vi "svx_Channel Type to Sensor Type String.vi"(3 "channel type":T1 items=["Voltage (V)"=0, "Charge (C)"=9, "-"=99, "SPL (Pa)"=3, "Force (lbf)"=6, "Force (N)"=1, "Acceleration (g) - IEPE"=2, "Acceleration (g) - Charge"=12, "Acceleration (g) - 4 wire DC Voltage"=22, "Velocity (in/s)"=7, "Velocity (mm/s)"=8, "Prox Probe (mil)"=4, "Prox Probe (mm)"=5]) -> (1 "sensor type":string)   [LabVIEW 2017, in "SVX NI-DAQmx AI Configuration XControl.xctl"]
uses:
  <vilib>/addons/Sound and Vibration/svt_DAQmx/Configuration XControl/SVX NI-DAQmx AI Configuration XControl.xctl
  <vilib>/addons/Sound and Vibration/svt_DAQmx/Configuration XControl/Controls/svx_DAQ_ChannelType.ctl
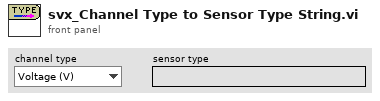
[diagram p1: front panel]
types:
  T1 = typedef "SVX NI-DAQmx AI Configuration XControl.xctl/svx_DAQ_ChannelType.ctl" = u16
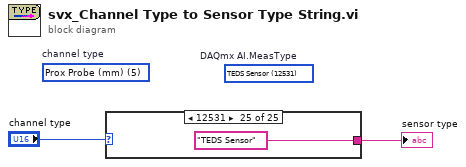
[diagram p0: block diagram]
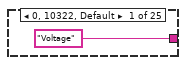
[diagram p2: hidden frame]
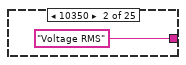
[diagram p3: hidden frame]
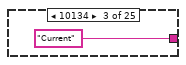
[diagram p4: hidden frame]
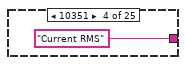
[diagram p5: hidden frame]
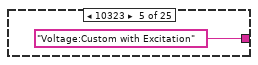
[diagram p6: hidden frame]
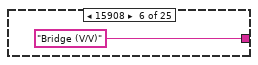
[diagram p7: hidden frame]
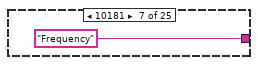
[diagram p8: hidden frame]
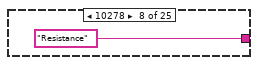
[diagram p9: hidden frame]
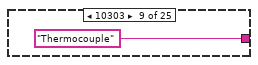
[diagram p10: hidden frame]
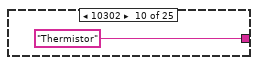
[diagram p11: hidden frame]
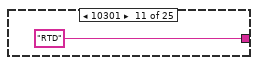
[diagram p12: hidden frame]
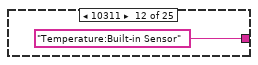
[diagram p13: hidden frame]
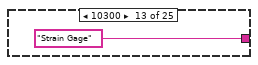
[diagram p14: hidden frame]
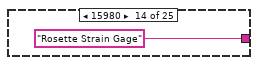
[diagram p15: hidden frame]
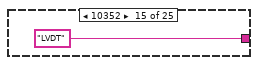
[diagram p16: hidden frame]
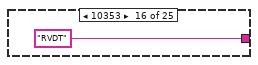
[diagram p17: hidden frame]
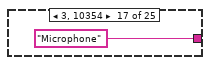
[diagram p18: hidden frame]
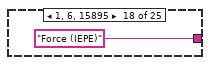
[diagram p19: hidden frame]
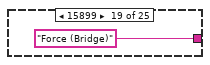
[diagram p20: hidden frame]
diagram:
  (unwired) T1 5 items=["Voltage (V)"=0, "SPL (Pa)"=3, "Force (lbf)"=6, "Force (N)"=1, "Acceleration (g)"=2, "Velocity (in/s)"=7, "Velocity (mm/s)"=8, "Prox Probe (mil)"=4, "Prox Probe (mm)"=5]  # channel type
  (unwired) 12531 items=["Voltage"=10322, "Voltage RMS"=10350, "Current"=10134, "Current RMS"=10351, "More:Voltage:Custom with Excitation"=10323, "More:Bridge (V/V)"=15908, "Frequency"=10181, "Resistance"=10278, "Temperature:Thermocouple"=10303, "Temperature:Thermistor"=10302, "Temperature:RTD"=10301, "Temperature:Built-in Sensor"=10311, "Strain Gage"=10300, "Rosette Strain Gage"=15980, "Position:LVDT"=10352, "Position:RVDT"=10353, "Position:Eddy Current Proximity Probe"=14835, "Accelerometer"=10356, "Velocity:IEPE Sensor"=15966, "Force:Bridge"=15899, "Force:IEPE Sensor"=15895, "Pressure:Bridge"=15902, "Sound Pressure:Microphone"=10354, "Torque:Bridge"=15905, "TEDS Sensor"=12531]  # DAQmx AI.MeasType
  n1 = case shown="12531" "channel type" {
    tunnel: ["Voltage" "Voltage RMS" "Current" "Current RMS" "Voltage:Custom with Excitation" "Bridge (V/V)" "Frequency" "Resistance" "Thermocouple" "Thermistor" "RTD" "Temperature:Built-in Sensor" "Strain Gage" "Rosette Strain Gage" "LVDT" "RVDT" "Microphone" "Force (IEPE)" "Force (Bridge)" "Pressure (Bridge)" "Torque (Bridge)" "Accelerometer" "Velocity (IEPE)" "Proximity Probe" "TEDS Sensor"] -> w2
    frame 0, 10322, Default {
    }
    frame 10350 {
    }
    frame 10134 {
    }
    frame 10351 {
    }
    frame 10323 {
    }
    frame 15908 {
    }
    frame 10181 {
    }
    frame 10278 {
    }
    frame 10303 {
    }
    frame 10302 {
    }
    frame 10301 {
    }
    frame 10311 {
    }
    frame 10300 {
    }
    frame 15980 {
    }
    frame 10352 {
    }
    frame 10353 {
    }
    frame 3, 10354 {
    }
    frame 1, 6, 15895 {
    }
    frame 15899 {
    }
    frame 15902 {
    }
    frame 15905 {
    }
    frame 2, 10356 {
    }
    frame 7, 8, 15966 {
    }
    frame 4, 5, 14835 {
    }
    frame 12531 {
    }
  }
  "sensor type" <- w2
